vi "ALARMS.vi"(8 "Error In":errorcluster, 10 "ALARM Input":bool[](array[boolean]), 11 "PROC OK Input":bool[](array[boolean])) -> (0 "Error Out":errorcluster, 2 "ALARM Output":bool[](array[boolean]), 3 "PROC OK Output":bool[](array[boolean]))   [LabVIEW 2023, in "QSM - Alarms.lvlib"]
uses:
  QSM - Alarms.lvlib
  Controls/State Machine Message.ctl
  Controls/Message Queue Element Position.ctl
  Controls/Event Handler Message.ctl
  <vilib>/event_ctls.llb/usereventprio.ctl
  QSM - Main/QSM - Main.lvlib
  Controls/procnokstr.ctl
  Controls/procnokLED.ctl
  Controls/procnokLEDScontrol.ctl
  Controls/procnokstringscontrol.ctl
  Controls/alarmstr.ctl
  Controls/Alarmstringscontrol.ctl
  Controls/AlarmLED.ctl
  Controls/AlarmLEDscontrol.ctl
panel:
  out "ALARM LED":bool
  in  "Clear ALARMS":bool
  out "ALARMS":T1
  in  "Alarm strings":T3
  in  "MAIN Page":bool
  out "PROC NOK LED":bool
  in  "CLEAR PROCNOK":bool
  out "PROCNOK":T5
  in  "PROCNOK strings":T7
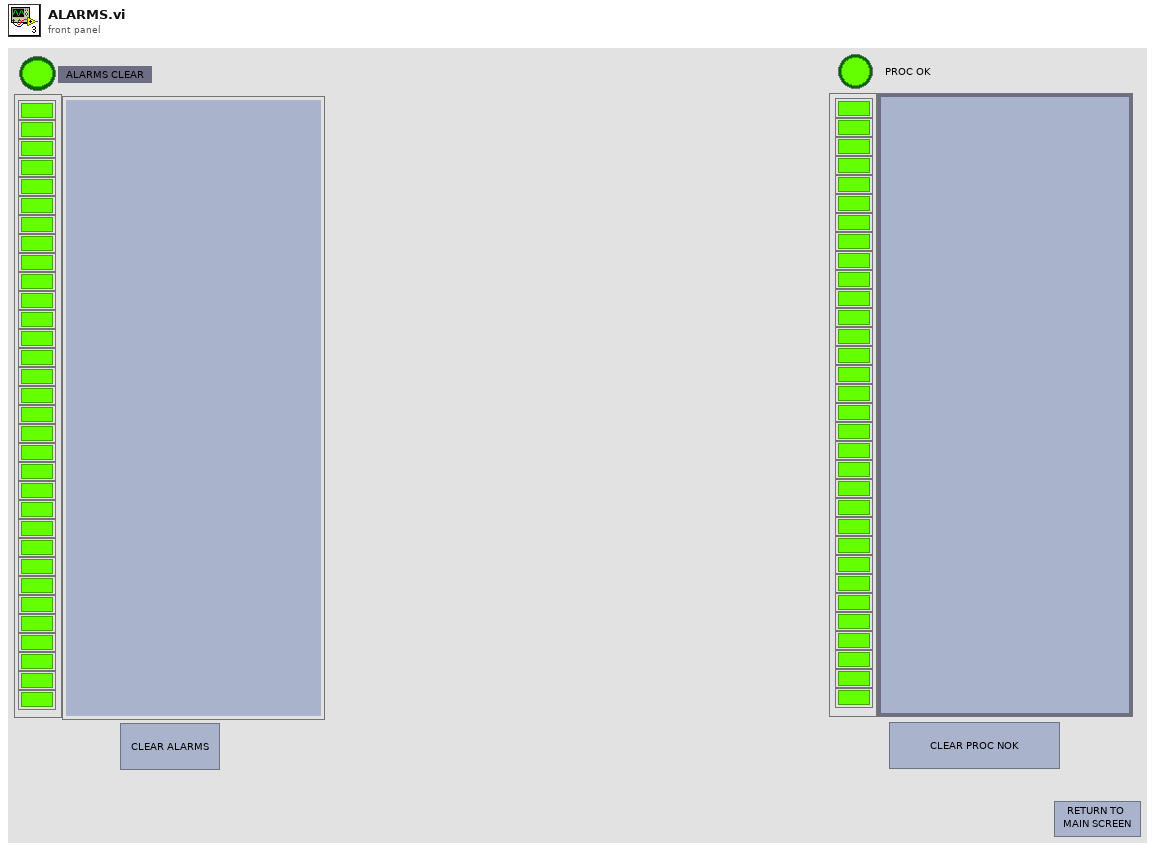
[diagram p1: front panel]
types:
  T1 = typedef "QSM - Alarms.lvlib/AlarmLEDscontrol.ctl" = cluster{"ALARM LIGHT":T2, "ALARM LIGHT 2":T2, "ALARM LIGHT 3":T2, "ALARM LIGHT 4":T2, "ALARM LIGHT 5":T2, "ALARM LIGHT 6":T2, "ALARM LIGHT 7":T2, "ALARM LIGHT 8":T2, "ALARM LIGHT 9":T2, "ALARM LIGHT 10":T2, "ALARM LIGHT 11":T2, "ALARM LIGHT 12":T2, "ALARM LIGHT 13":T2, "ALARM LIGHT 14":T2, "ALARM LIGHT 15":T2, "ALARM LIGHT 16":T2, "ALARM LIGHT 17":T2, "ALARM LIGHT 18":T2, "ALARM LIGHT 19":T2, "ALARM LIGHT 20":T2, "ALARM LIGHT 21":T2, "ALARM LIGHT 22":T2, "ALARM LIGHT 23":T2, "ALARM LIGHT 24":T2, "ALARM LIGHT 25":T2, "ALARM LIGHT 26":T2, "ALARM LIGHT 27":T2, "ALARM LIGHT 28":T2, "ALARM LIGHT 29":T2, "ALARM LIGHT 30":T2, "ALARM LIGHT 31":T2, "ALARM LIGHT 32":T2}
  T2 = typedef "QSM - Alarms.lvlib/AlarmLED.ctl" = bool
  T3 = typedef "QSM - Alarms.lvlib/Alarmstringscontrol.ctl" = cluster{"Alarm str":T4, "Alarm str 2":T4, "Alarm str 3":T4, "Alarm str 4":T4, "Alarm str 5":T4, "Alarm str 6":T4, "Alarm str 7":T4, "Alarm str 8":T4, "Alarm str 9":T4, "Alarm str 10":T4, "Alarm str 11":T4, "Alarm str 12":T4, "Alarm str 13":T4, "Alarm str 14":T4, "Alarm str 15":T4, "Alarm str 16":T4, "Alarm str 17":T4, "Alarm str 18":T4, "Alarm str 19":T4, "Alarm str 20":T4, "Alarm str 21":T4, "Alarm str 22":T4, "Alarm str 23":T4, "Alarm str 24":T4, "Alarm str 25":T4, "Alarm str 26":T4, "Alarm str 27":T4, "Alarm str 28":T4, "Alarm str 29":T4, "Alarm str 30":T4, "Alarm str 31":T4, "Alarm str 32":T4}
  T4 = typedef "QSM - Alarms.lvlib/alarmstr.ctl" = string
  T5 = typedef "QSM - Alarms.lvlib/procnokLEDScontrol.ctl" = cluster{"PROCNOK":T6, "PROCNOK 2":T6, "PROCNOK 3":T6, "PROCNOK 4":T6, "PROCNOK 5":T6, "PROCNOK 6":T6, "PROCNOK 7":T6, "PROCNOK 8":T6, "PROCNOK 9":T6, "PROCNOK 10":T6, "PROCNOK 11":T6, "PROCNOK 12":T6, "PROCNOK 13":T6, "PROCNOK 14":T6, "PROCNOK 15":T6, "PROCNOK 16":T6, "PROCNOK 17":T6, "PROCNOK 18":T6, "PROCNOK 19":T6, "PROCNOK 20":T6, "PROCNOK 21":T6, "PROCNOK 22":T6, "PROCNOK 23":T6, "PROCNOK 24":T6, "PROCNOK 25":T6, "PROCNOK 26":T6, "PROCNOK 27":T6, "PROCNOK 28":T6, "PROCNOK 29":T6, "PROCNOK 30":T6, "PROCNOK 31":T6, "PROCNOK 32":T6}
  T6 = typedef "QSM - Alarms.lvlib/procnokLED.ctl" = bool
  T7 = typedef "QSM - Alarms.lvlib/procnokstringscontrol.ctl" = cluster{"PROCNOKSTR":T8, "PROCNOKSTR 2":T8, "PROCNOKSTR 3":T8, "PROCNOKSTR 4":T8, "PROCNOKSTR 5":T8, "PROCNOKSTR 6":T8, "PROCNOKSTR 7":T8, "PROCNOKSTR 8":T8, "PROCNOKSTR 9":T8, "PROCNOKSTR 10":T8, "PROCNOKSTR 11":T8, "PROCNOKSTR 12":T8, "PROCNOKSTR 13":T8, "PROCNOKSTR 14":T8, "PROCNOKSTR 15":T8, "PROCNOKSTR 16":T8, "PROCNOKSTR 17":T8, "PROCNOKSTR 18":T8, "PROCNOKSTR 19":T8, "PROCNOKSTR 20":T8, "PROCNOKSTR 21":T8, "PROCNOKSTR 22":T8, "PROCNOKSTR 23":T8, "PROCNOKSTR 24":T8, "PROCNOKSTR 25":T8, "PROCNOKSTR 26":T8, "PROCNOKSTR 27":T8, "PROCNOKSTR 28":T8, "PROCNOKSTR 29":T8, "PROCNOKSTR 30":T8, "PROCNOKSTR 31":T8, "PROCNOKSTR 32":T8}
  T8 = typedef "QSM - Alarms.lvlib/procnokstr.ctl" = string
  T9 = typedef "QSM - Alarms.lvlib/State Machine Message.ctl" = enum16{"Initialize", "PROC OK Change", "Get Main PROCNOK", "CLEAR PROC NOK", "ALARM SET", "CLEAR ALARMS", "CHECKS", "Handle Error", "Exit"}
  T10 = typedef "QSM - Alarms.lvlib/User Event Reference.ctl" = refnum<user-event>
  T11 = typedef "QSM - Alarms.lvlib/User Event Registration Reference.ctl" = refnum<event-registration>
  T12 = typedef "QSM - Alarms.lvlib/Message Queue Element Position.ctl" = enum16{"Front", "Back"}
  T13 = typedef "QSM - Alarms.lvlib/Event Handler Message.ctl" = enum16{"Exit"}
  T14 = typedef "usereventprio.ctl" = enum32{"high priority", "normal priority"}
  T15 = cluster{"Value[0]":bool, "Value[1]":bool, "Value[2]":bool, "Value[3]":bool, "Value[4]":bool, "Value[5]":bool, "Value[6]":bool, "Value[7]":bool, "Value[8]":bool, "Value[9]":bool, "Value[10]":bool, "Value[11]":bool, "Value[12]":bool, "Value[13]":bool, "Value[14]":bool, "Value[15]":bool, "Value[16]":bool, "Value[17]":bool, "Value[18]":bool, "Value[19]":bool, "Value[20]":bool, "Value[21]":bool, "Value[22]":bool, "Value[23]":bool, "Value[24]":bool, "Value[25]":bool, "Value[26]":bool, "Value[27]":bool, "Value[28]":bool, "Value[29]":bool, "Value[30]":bool, "Value[31]":bool}
  T16 = cluster{"[0]":bool, "[1]":bool, "[2]":bool, "[3]":bool, "[4]":bool, "[5]":bool, "[6]":bool, "[7]":bool, "[8]":bool, "[9]":bool, "[10]":bool, "[11]":bool, "[12]":bool, "[13]":bool, "[14]":bool, "[15]":bool, "[16]":bool, "[17]":bool, "[18]":bool, "[19]":bool, "[20]":bool, "[21]":bool, "[22]":bool, "[23]":bool, "[24]":bool, "[25]":bool, "[26]":bool, "[27]":bool, "[28]":bool, "[29]":bool, "[30]":bool, "[31]":bool}
  T17 = cluster{"[0]":T6, "[1]":T6, "[2]":T6, "[3]":T6, "[4]":T6, "[5]":T6, "[6]":T6, "[7]":T6, "[8]":T6, "[9]":T6, "[10]":T6, "[11]":T6, "[12]":T6, "[13]":T6, "[14]":T6, "[15]":T6, "[16]":T6, "[17]":T6, "[18]":T6, "[19]":T6, "[20]":T6, "[21]":T6, "[22]":T6, "[23]":T6, "[24]":T6, "[25]":T6, "[26]":T6, "[27]":T6, "[28]":T6, "[29]":T6, "[30]":T6, "[31]":T6}
  T18 = cluster{"ALARM LIGHT":T2, "ALARM LIGHT 2":T2, "ALARM LIGHT 3":T2, "ALARM LIGHT 4":T2, "ALARM LIGHT 5":T2, "ALARM LIGHT 6":T2, "ALARM LIGHT 7":T2, "ALARM LIGHT 8":T2, "ALARM LIGHT 9":T2, "ALARM LIGHT 10":T2, "ALARM LIGHT 11":T2, "ALARM LIGHT 12":T2, "ALARM LIGHT 13":T2, "ALARM LIGHT 14":T2, "ALARM LIGHT 15":T2, "ALARM LIGHT 16":T2, "ALARM LIGHT 17":T2, "ALARM LIGHT 18":T2, "ALARM LIGHT 19":T2, "ALARM LIGHT 20":T2, "ALARM LIGHT 21":T2, "ALARM LIGHT 22":T2, "ALARM LIGHT 23":T2, "ALARM LIGHT 24":T2, "ALARM LIGHT 25":T2, "ALARM LIGHT 26":T2, "ALARM LIGHT 27":T2, "ALARM LIGHT 28":T2, "ALARM LIGHT 29":T2, "ALARM LIGHT 30":T2, "ALARM LIGHT 31":T2, "ALARM LIGHT 32":T2}
  T19 = cluster{"Value[0]":T2, "Value[1]":T2, "Value[2]":T2, "Value[3]":T2, "Value[4]":T2, "Value[5]":T2, "Value[6]":T2, "Value[7]":T2, "Value[8]":T2, "Value[9]":T2, "Value[10]":T2, "Value[11]":T2, "Value[12]":T2, "Value[13]":T2, "Value[14]":T2, "Value[15]":T2, "Value[16]":T2, "Value[17]":T2, "Value[18]":T2, "Value[19]":T2, "Value[20]":T2, "Value[21]":T2, "Value[22]":T2, "Value[23]":T2, "Value[24]":T2, "Value[25]":T2, "Value[26]":T2, "Value[27]":T2, "Value[28]":T2, "Value[29]":T2, "Value[30]":T2, "Value[31]":T2}
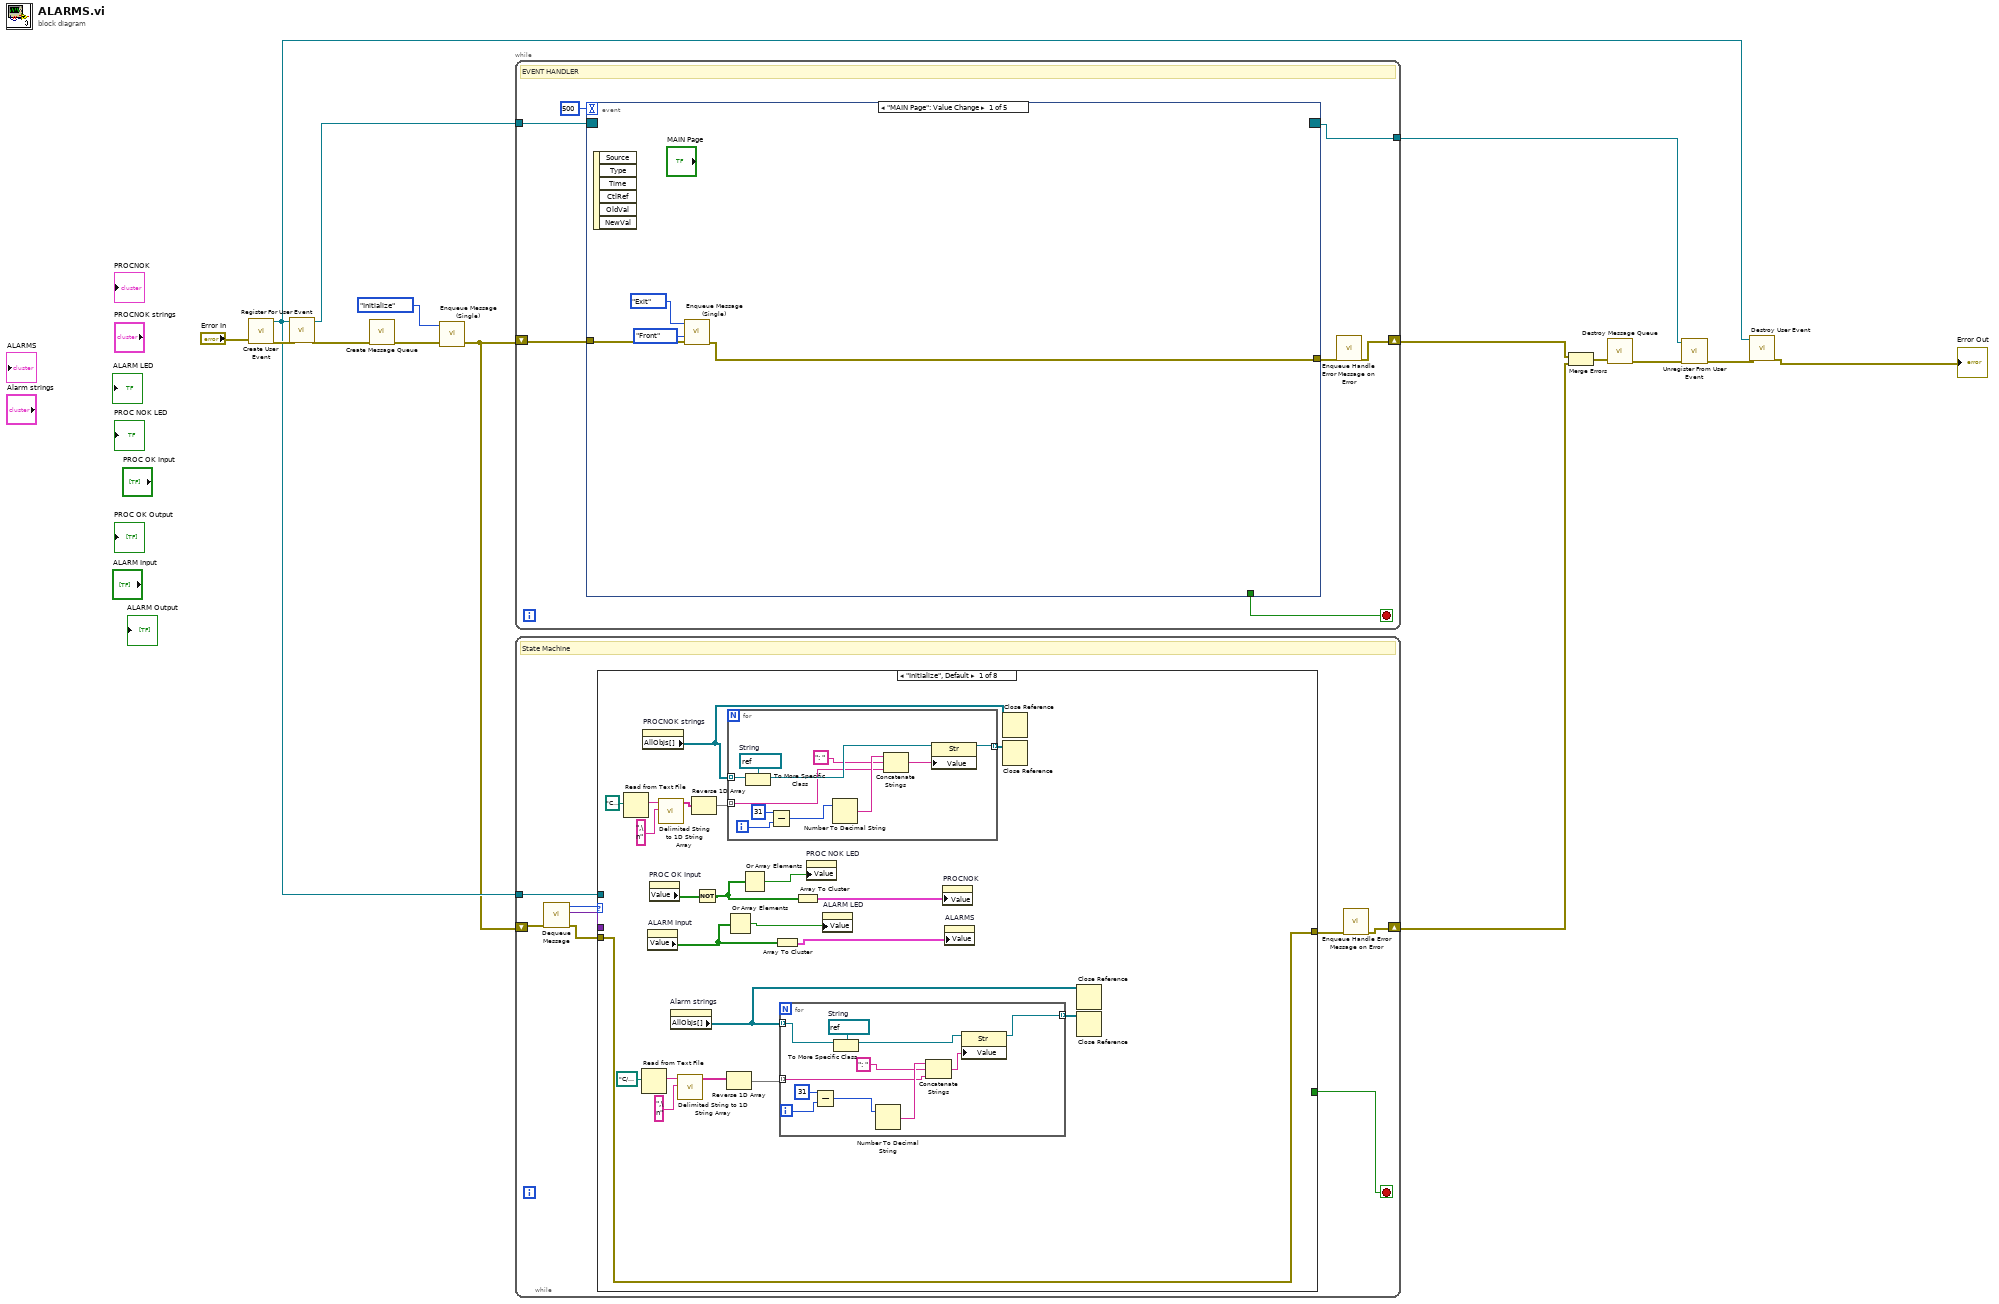
[diagram p0: block diagram]
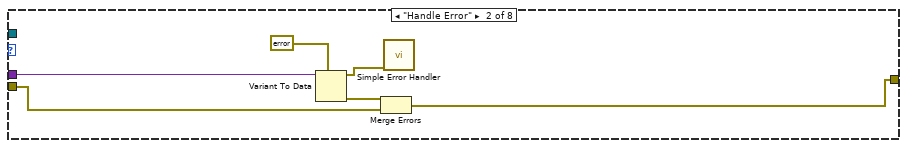
[diagram p2: hidden frame]
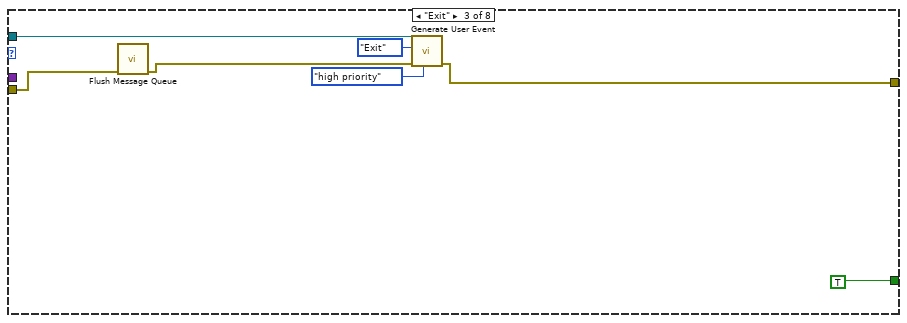
[diagram p3: hidden frame]
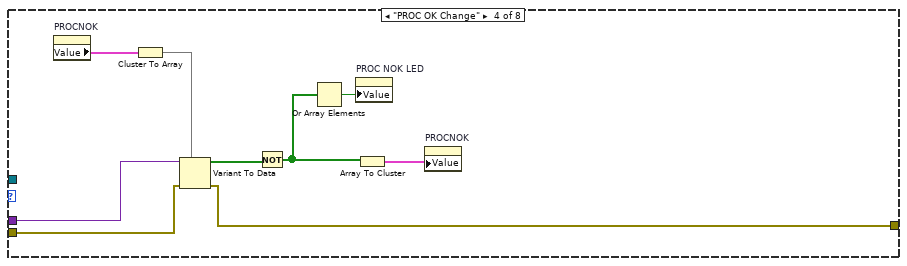
[diagram p4: hidden frame]
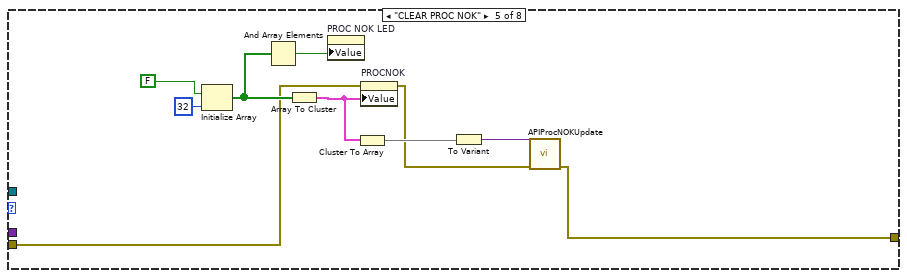
[diagram p5: hidden frame]
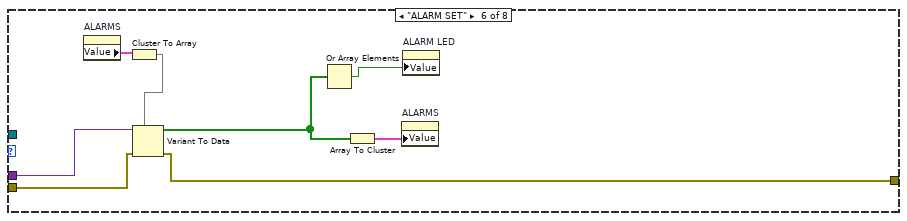
[diagram p6: hidden frame]
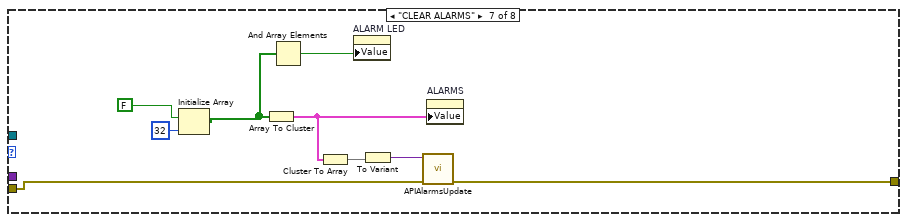
[diagram p7: hidden frame]
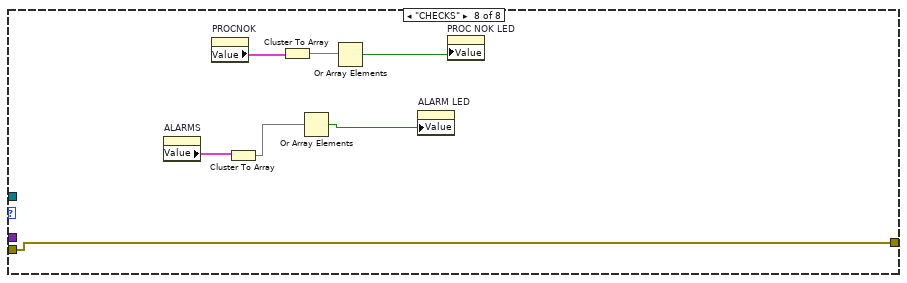
[diagram p8: hidden frame]
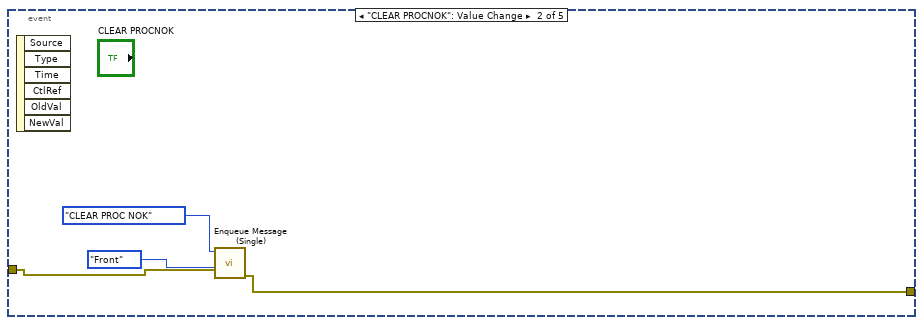
[diagram p9: hidden frame]
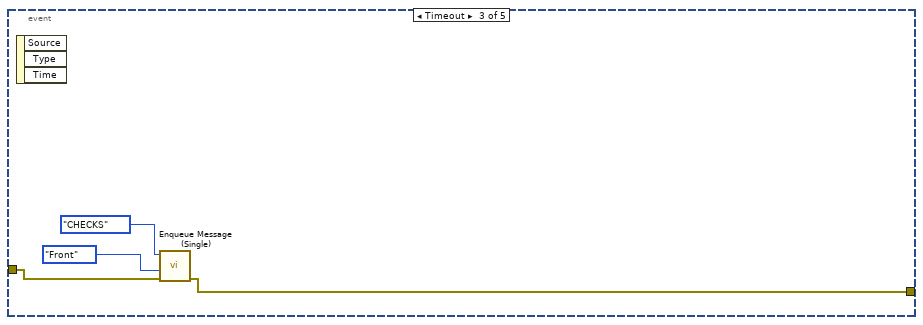
[diagram p10: hidden frame]
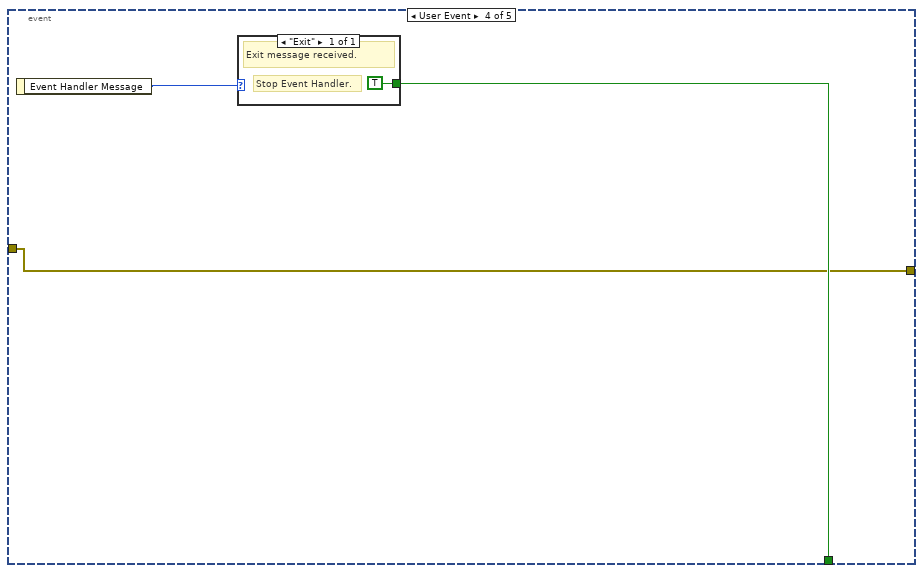
[diagram p11: hidden frame]
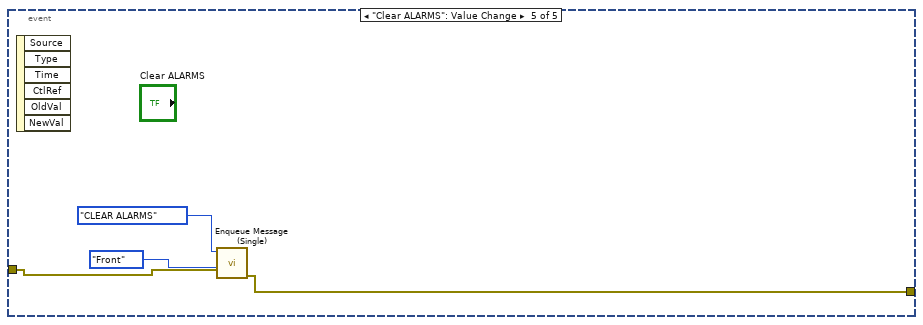
[diagram p12: hidden frame]
diagram:
  n1 = call "Create User Event.vi"("Error In"="Error In") -> ("Error Out"=w13:errorcluster, "User Event Reference"=w3:T10)  [unwired: 9 in]
  n2 = call "Register For User Event.vi"("Error In"=w13, "User Event Reference"=w3) -> ("Error Out"=w9:errorcluster, "User Event Registration Reference"=w7:T11)  [unwired: 8 in]
  n3 = call "Create Message Queue.vi"("Error In"=w9) -> ("Error Out"=w1:errorcluster)  [unwired: 10 in]
  n4 = call "Enqueue Message (Single).vi"("State Machine Message"=State_Machine_Message."Initialize") -> ()  [unwired: 10 in, 1 out]
  n5 = while {
    shift-right: [w20] -> w11
    shift-left: w1 -> [w21]
    tunnel: w7 -> [w15]
    tunnel: [w16] -> w2
    stop <- w18 stop-if-true
    # "EVENT HANDLER"
    n6 = event shown="[0] \"MAIN Page\": Value Change" {
      selector: w15 -> [_ _ _ _ _]
      dyn-events: [_ _ _ _ _] -> w16
      timeout: 500 -> [_ _ _ _ _]
      tunnel: w21 -> [w25 w27 w31 w34 w39]
      tunnel: [w22 w26 w30 w34 w38] -> w19
      tunnel: [_ _ _ w35 _] -> w18
      event "MAIN Page": Value Change {
        n7 = event-data() -> ()  [unwired: 1 in, 6 out]
        n8 = call "Enqueue Message (Single).vi"("Error In"=w25, "Message Position"=Message_Queue_Element_Position."Front", "State Machine Message"=State_Machine_Message."Exit") -> ("Error Out"=w22:errorcluster)  [unwired: 8 in]
      }
      event "CLEAR PROCNOK": Value Change {
        n9 = event-data() -> ()  [unwired: 1 in, 6 out]
        n10 = call "Enqueue Message (Single).vi"("Error In"=w27, "Message Position"=Message_Queue_Element_Position."Front", "State Machine Message"=State_Machine_Message."CLEAR PROC NOK") -> ("Error Out"=w26:errorcluster)  [unwired: 8 in]
      }
      event Timeout {
        n11 = event-data() -> ()  [unwired: 1 in, 3 out]
        n12 = call "Enqueue Message (Single).vi"("Error In"=w31, "Message Position"=Message_Queue_Element_Position."Front", "State Machine Message"=State_Machine_Message."CHECKS") -> ("Error Out"=w30:errorcluster)  [unwired: 8 in]
      }
      event User Event {
        n13 = event-data() -> ("Event Handler Message"=w36:T13)  [unwired: 1 in]
        n14 = case shown="\"Exit\"" w36 {
          tunnel: [TRUE] -> w35
          frame "Exit" {
            # "Stop Event Handler."
            # "Exit message received."
          }
        }
      }
      event "Clear ALARMS": Value Change {
        n15 = event-data() -> ()  [unwired: 1 in, 6 out]
        n16 = call "Enqueue Message (Single).vi"("Error In"=w39, "Message Position"=Message_Queue_Element_Position."Front", "State Machine Message"=State_Machine_Message."CLEAR ALARMS") -> ("Error Out"=w38:errorcluster)  [unwired: 8 in]
      }
    }
    n17 = call "Enqueue Handle Error Message on Error.vi"("Error In"=w19) -> ("Error Out"=w20:errorcluster)  [unwired: 10 in]
  }
  n18 = while {
    shift-right: [w49] -> w10
    shift-left: w1 -> [w48]
    tunnel: w3 -> [w42]
    stop <- w43 stop-if-true
    # "State Machine"
    n19 = call "Dequeue Message.vi"("Error In"=w48) -> ("Error Out"=w46:errorcluster, "Data"=w44:variant, "State Machine Message"=w47:T9)  [unwired: 8 in]
    n20 = case shown="\"Initialize\", Default" w47 {
      tunnel: w46 -> [w71 w96 w106 w110 w121 w131 w139 w149]
      tunnel: [w71 w94 w103 w109 w116 w130 w138 w149] -> w45
      tunnel: w44 -> [_ w95 _ w115 _ w132 _ _]
      tunnel: [_ _ TRUE _ _ _ _ _] -> w43
      tunnel: w42 -> [_ _ w102 _ _ _ _ _]
      frame "Initialize", Default {
        n21 = Read from Text File(file (use dialog)=path "C:/Users/Public/Documents/Grid2093/ALARMS/PROCNOK.txt") -> (text=w68:string)  [unwired: 3 in, 3 out]
        n22 = Read from Text File(file (use dialog)=path "C:/Users/Public/Documents/Grid2093/ALARMS/ALARMS.txt") -> (text=w59:string)  [unwired: 3 in, 3 out]
        n23 = property on="PROCNOK strings" class="Clust (strict)"() -> ("AllObjs[]"=w70:refnum<vi>[])  [unwired: 2 in, 2 out]
        n24 = property on="ALARM Input" class="Arr (strict)"() -> ("Value"=w56:bool[])  [unwired: 2 in, 2 out]
        n25 = property on="PROC OK Input" class="Arr (strict)"() -> ("Value"=w64:bool[])  [unwired: 2 in, 2 out]
        n26 = call <vilib>:"Delimited String to 1D String Array.vi"("delimiter"=",\n", "delimited string"=w68) -> ("string array"=w53:string[])  [unwired: 9 in]
        n27 = property on="Alarm strings" class="Clust (strict)"() -> ("AllObjs[]"=w58:refnum<vi>[])  [unwired: 2 in, 2 out]
        n28 = call <vilib>:"Delimited String to 1D String Array.vi"("delimiter"=",\n", "delimited string"=w59) -> ("string array"=w51:string[])  [unwired: 9 in]
        n29 = Reverse 1D Array(array=w53) -> (reversed array=w52:string[])
        n30 = Not(x=w64) -> (.not. x?=w62:bool[])
        n31 = Reverse 1D Array(array=w51) -> (reversed array=w50:string[])
        n32 = for {
          tunnel: [w91] -> w69 mode=indexing
          tunnel: w52 -> [w87] mode=indexing
          tunnel: w70 -> [w86] mode=indexing
          i -> [w84]
          w93 = refnum<vi> refnum  # String
          n33 = To More Specific Class(target class=w93, reference=w86) -> (specific class reference=w92:refnum<vi>)  [unwired: 1 in, 1 out]
          n34 = Subtract(x=31, y=w84) -> (x-y=w83:i32)
          n35 = Number To Decimal String(number=w83) -> (decimal integer string=w89:string)  [unwired: 1 in]
          n36 = Concatenate Strings(w89, ": " ("string"), w87) -> (w90:string)
          n37 = property class="Str"(reference=w92, "Value"=w90) -> (reference out=w91:refnum<vi>)  [unwired: 1 in, 1 out]
        }
        n38 = Or Array Elements(Boolean array=w56) -> (logical OR=w54:bool)
        n39 = Or Array Elements(Boolean array=w62) -> (logical OR=w63:bool)
        n40 = Array To Cluster(array=w56) -> (cluster=w55:T15)
        n41 = for {
          tunnel: w50 -> [w78] mode=indexing
          tunnel: w58 -> [w82] mode=indexing
          tunnel: [w75] -> w57 mode=indexing
          i -> [w73]
          w81 = refnum<vi> refnum  # String
          n42 = Subtract(x=31, y=w73) -> (x-y=w72:i32)
          n43 = To More Specific Class(target class=w81, reference=w82) -> (specific class reference=w76:refnum<vi>)  [unwired: 1 in, 1 out]
          n44 = Number To Decimal String(number=w72) -> (decimal integer string=w80:string)  [unwired: 1 in]
          n45 = Concatenate Strings(w80, ": " ("string"), w78) -> (w77:string)
          n46 = property class="Str"(reference=w76, "Value"=w77) -> (reference out=w75:refnum<vi>)  [unwired: 1 in, 1 out]
        }
        n47 = Array To Cluster(array=w62) -> (cluster=w65:T16)
        n48 = property on="PROC NOK LED" class="Bool (strict)"("Value"=w63) -> ()  [unwired: 2 in, 2 out]
        n49 = property on="ALARM LED" class="Bool (strict)"("Value"=w54) -> ()  [unwired: 2 in, 2 out]
        n50 = property on="PROCNOK" class="Clust (strict)"("Value"=w65) -> ()  [unwired: 2 in, 2 out]
        n51 = property on="ALARMS" class="Clust (strict)"("Value"=w55) -> ()  [unwired: 2 in, 2 out]
        n52 = Close Reference(reference=w69) -> ()  [unwired: 1 in, 1 out]
        n53 = Close Reference(reference=w70) -> ()  [unwired: 1 in, 1 out]
        n54 = Close Reference(reference=w58) -> ()  [unwired: 1 in, 1 out]
        n55 = Close Reference(reference=w57) -> ()  [unwired: 1 in, 1 out]
      }
      frame "Handle Error" {
        n56 = Variant To Data(type=errorcluster {"status"=FALSE, "code"=0, "source"=""} ("Error In"), Variant=w95) -> (data=w97:errorcluster, error out=w98:errorcluster)  [unwired: 1 in]
        n57 = Merge Errors(w98, w96) -> (w94:errorcluster)
        n58 = call <vilib>:"Simple Error Handler.vi"("error in (no error)"=w97) -> ()  [unwired: 4 in, 5 out]
      }
      frame "Exit" {
        n59 = call "Flush Message Queue.vi"("Error In"=w106) -> ("Error Out"=w104:errorcluster)  [unwired: 9 in, 1 out]
        n60 = call "Generate User Event.vi"("User Event Priority"=usereventprio."high priority", "Error In"=w104, "Event Handler Message"=Event_Handler_Message."Exit", "User Event Reference"=w102) -> ("Error Out"=w103:errorcluster)  [unwired: 7 in]
      }
      frame "PROC OK Change" {
        n61 = property on="PROCNOK" class="Clust (strict)"() -> ("Value"=w114:T5)  [unwired: 2 in, 2 out]
        n62 = Cluster To Array(cluster=w114) -> (array=w113:T6[])
        n63 = Variant To Data(error in=w110, type=w113, Variant=w115) -> (data=w108:T6[], error out=w109:errorcluster)
        n64 = Not(x=w108) -> (.not. x?=w107:T6[])
        n65 = Or Array Elements(Boolean array=w107) -> (logical OR=w111:bool)
        n66 = property on="PROC NOK LED" class="Bool (strict)"("Value"=w111) -> ()  [unwired: 2 in, 2 out]
        n67 = Array To Cluster(array=w107) -> (cluster=w112:T17)
        n68 = property on="PROCNOK" class="Clust (strict)"("Value"=w112) -> ()  [unwired: 2 in, 2 out]
      }
      frame "CLEAR PROC NOK" {
        n69 = Initialize Array(FALSE, 32 ("dimension size")) -> (w123:bool[])
        n70 = And Array Elements(Boolean array=w123) -> (logical AND=w122:bool)
        n71 = Array To Cluster(array=w123) -> (cluster=w119:T16)
        n72 = property on="PROC NOK LED" class="Bool (strict)"("Value"=w122) -> ()  [unwired: 2 in, 2 out]
        n73 = Cluster To Array(cluster=w119) -> (array=w118:bool[])
        n74 = property on="PROCNOK" class="Clust (strict)"(error in=w121, "Value"=w119) -> (error out=w117:errorcluster)  [unwired: 1 in, 1 out]
        n75 = To Variant(anything=w118) -> (Variant=w120:variant)
        n76 = call "APIProcNOKUpdate.vi"("Error In"=w117, "Data"=w120) -> ("Error Out"=w116:errorcluster)  [unwired: 9 in]
      }
      frame "ALARM SET" {
        n77 = property on="ALARMS" class="Clust (strict)"() -> ("Value"=w129:T18)  [unwired: 2 in, 2 out]
        n78 = Cluster To Array(cluster=w129) -> (array=w128:T2[])
        n79 = Variant To Data(error in=w131, type=w128, Variant=w132) -> (data=w127:T2[], error out=w130:errorcluster)
        n80 = Or Array Elements(Boolean array=w127) -> (logical OR=w133:bool)
        n81 = Array To Cluster(array=w127) -> (cluster=w126:T19)
        n82 = property on="ALARMS" class="Clust (strict)"("Value"=w126) -> ()  [unwired: 2 in, 2 out]
        n83 = property on="ALARM LED" class="Bool (strict)"("Value"=w133) -> ()  [unwired: 2 in, 2 out]
      }
      frame "CLEAR ALARMS" {
        n84 = Initialize Array(FALSE, 32 ("dimension size")) -> (w137:bool[])
        n85 = Array To Cluster(array=w137) -> (cluster=w135:T16)
        n86 = And Array Elements(Boolean array=w137) -> (logical AND=w140:bool)
        n87 = Cluster To Array(cluster=w135) -> (array=w134:bool[])
        n88 = property on="ALARM LED" class="Bool (strict)"("Value"=w140) -> ()  [unwired: 2 in, 2 out]
        n89 = To Variant(anything=w134) -> (Variant=w136:variant)
        n90 = call "APIAlarmsUpdate.vi"("Error In"=w139, "Data"=w136) -> ("Error Out"=w138:errorcluster)  [unwired: 9 in]
        n91 = property on="ALARMS" class="Clust (strict)"("Value"=w135) -> ()  [unwired: 2 in, 2 out]
      }
      frame "CHECKS" {
        n92 = property on="ALARMS" class="Clust (strict)"() -> ("Value"=w144:T1)  [unwired: 2 in, 2 out]
        n93 = property on="PROCNOK" class="Clust (strict)"() -> ("Value"=w148:T5)  [unwired: 2 in, 2 out]
        n94 = Cluster To Array(cluster=w144) -> (array=w143:T2[])
        n95 = Cluster To Array(cluster=w148) -> (array=w147:T6[])
        n96 = Or Array Elements(Boolean array=w143) -> (logical OR=w145:bool)
        n97 = Or Array Elements(Boolean array=w147) -> (logical OR=w146:bool)
        n98 = property on="ALARM LED" class="Bool (strict)"("Value"=w145) -> ()  [unwired: 2 in, 2 out]
        n99 = property on="PROC NOK LED" class="Bool (strict)"("Value"=w146) -> ()  [unwired: 2 in, 2 out]
      }
    }
    n100 = call "Enqueue Handle Error Message on Error.vi"("Error In"=w45) -> ("Error Out"=w49:errorcluster)  [unwired: 10 in]
  }
  n101 = Merge Errors(w11, w10) -> (w12:errorcluster)
  n102 = call "Destroy Message Queue.vi"("Error In"=w12) -> ("Error Out"=w6:errorcluster)  [unwired: 10 in]
  n103 = call "Unregister From User Event.vi"("Error In"=w6, "User Event Registration Reference"=w2) -> ("Error Out"=w5:errorcluster)  [unwired: 9 in]
  n104 = call "Destroy User Event.vi"("Error In"=w5, "User Event Reference"=w3) -> ("Error Out"=→"Error Out":errorcluster)  [unwired: 9 in]
